vi "RAWFileLoadSample.vi"() -> ()   [LabVIEW 8.6]
panel:
  in  "Stop":bool
  out "Picture":picture
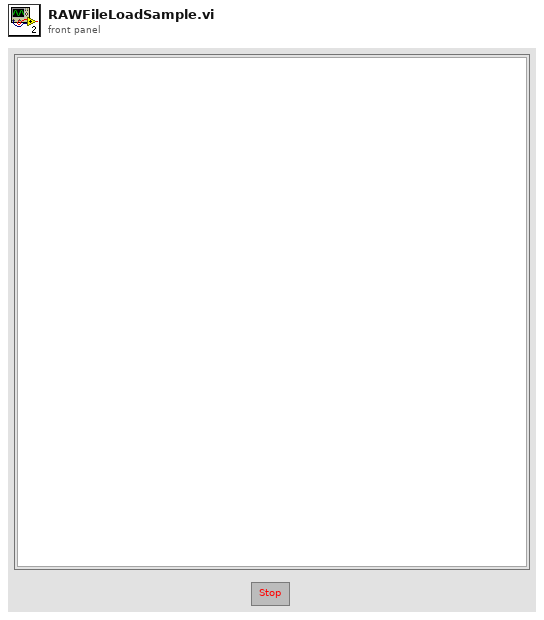
[diagram p1: front panel]
types:
  T1 = typedef "LVBoundsTypeDef.ctl" = cluster{"Width":u32, "Height":u32}
  T2 = cluster{"Width":i32, "Height":i32, "Byte Per Line":i32, "Real Bit Per Pixel":u16, "Interleave":i32}
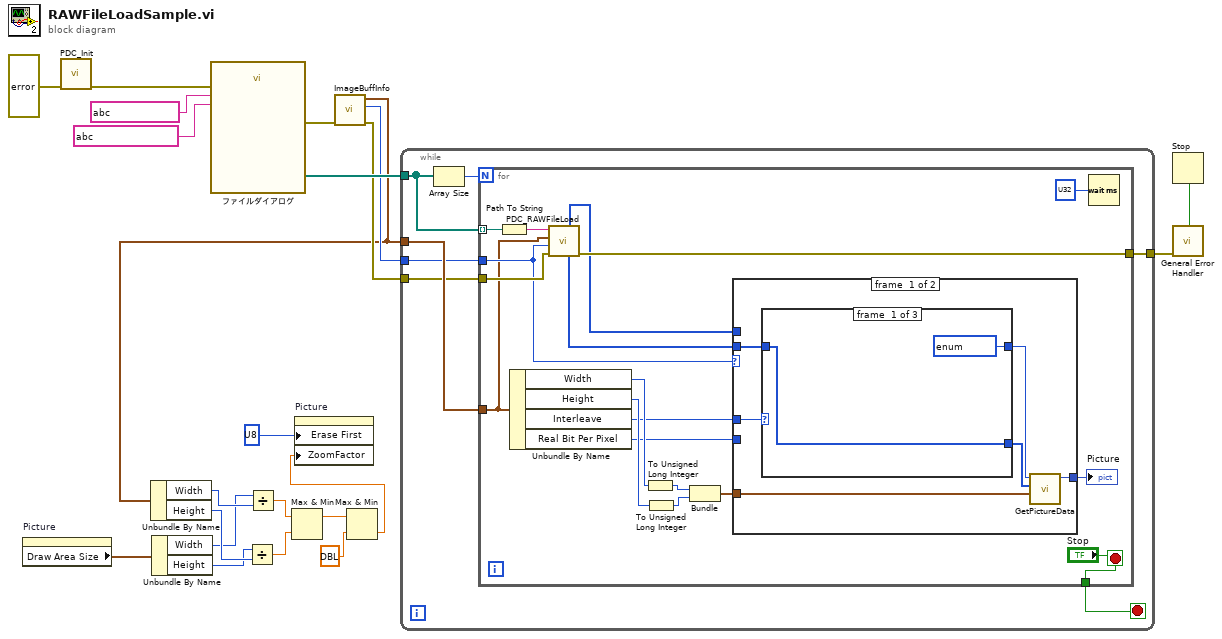
[diagram p0: block diagram]
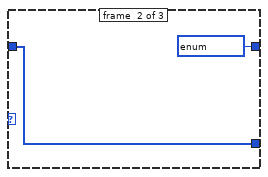
[diagram p2: hidden frame]
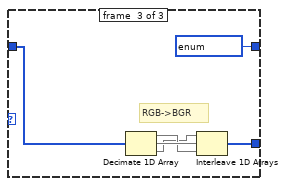
[diagram p3: hidden frame]
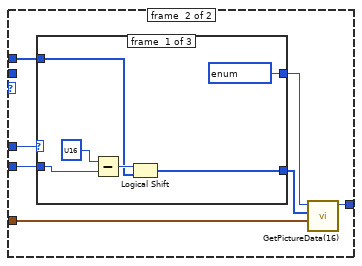
[diagram p4: hidden frame]
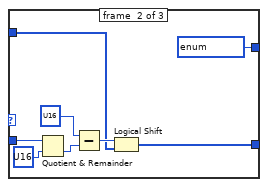
[diagram p5: hidden frame]
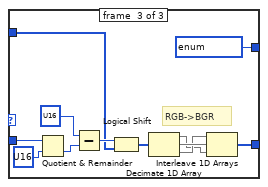
[diagram p6: hidden frame]
diagram:
  n1 = property on="Picture" class="Pict"() -> ("Draw Area Size"=w3:T1)  [unwired: 2 in, 2 out]
  n2 = call "PDC_Init.vi"("error in (no error)"=errorcluster ?) -> ("error out"=w19:errorcluster)  [unwired: 8 in, 2 out]
  n3 = Unbundle By Name(w3) -> ("Width"=w9:u32, "Height"=w8:u32)
  n4 = call "ファイルダイアログ"("error in"=w19, "pattern (all files)"=string ?, "pattern label"=string ?) -> ("selected paths"=w17:path[], "error out"=w16:errorcluster)  [unwired: 9 in, 2 out]
  n5 = call "ImageBuffInfo.vi"("error in (no error)"=w16) -> ("error out"=w14:errorcluster, "Raw Bit Depth"=w15:u32, "Image Buff Info"=w2:T2)  [unwired: 7 in, 1 out]
  n6 = Unbundle By Name(w2) -> ("Width"=w11:i32, "Height"=w10:i32)
  n7 = Divide(x=w8, y=w10) -> (x/y=w6:dbl)
  n8 = Divide(x=w9, y=w11) -> (x/y=w7:dbl)
  n9 = Max & Min(x=w7, y=w6) -> (max(x,y)=w5:dbl)  [unwired: 1 out]
  n10 = Max & Min(x=w5, y=dbl ?) -> (min(x,y)=w1:dbl)  [unwired: 1 out]
  n11 = property on="Picture" class="Pict"("Erase First"=u8 ? ("最初に削除"), "ZoomFactor"=w1) -> ()  [unwired: 2 in, 2 out]
  n12 = while {
    tunnel: w17 -> [w28]
    tunnel: w2 -> [w27]
    tunnel: w15 -> [w26]
    tunnel: w14 -> [w25]
    tunnel: [w24] -> w13
    stop <- w23 stop-if-true
    n13 = Array Size(array=w28) -> (size(s)=w29:i32)
    n14 = for {
      N: w29 -> [_]
      tunnel: w28 -> [w46] mode=indexing
      tunnel: w27 -> [w32]
      tunnel: w26 -> [w42]
      tunnel: w25 -> [w44]
      tunnel: [w43] -> w24
      tunnel: ["Stop"] -> w23
      stop <- "Stop" stop-if-true
      n15 = Path To String(path=w46) -> (string=w45:string)
      n16 = Unbundle By Name(w32) -> ("Width"=w37:i32, "Height"=w36:i32, "Interleave"=w31:i32, "Real Bit Per Pixel"=w30:u16)
      n17 = call "PDC_RAWFileLoad.vi"("FileName"=w45, "ImageBuffInfo"=w32, "RawBitDepth"=w42, "error in (no error)"=w44) -> ("Data(16Bit)"=w39:u16[], "Data(8Bit)"=w41:u8[], "error out"=w43:errorcluster)  [unwired: 2 in, 2 out]
      n18 = To Unsigned Long Integer(number=w37) -> (unsigned 32bit integer=w33:u32)
      n19 = To Unsigned Long Integer(number=w36) -> (unsigned 32bit integer=w35:u32)
      n20 = Bundle(w33, w35) -> (w38:cluster{u32, u32})  [unwired: 1 in]
      n21 = case shown="1..3, デフォルト" w42 {
        tunnel: w41 -> [w48 _]
        tunnel: [w52 w70] -> w40
        tunnel: w39 -> [_ w65]
        tunnel: w38 -> [w53 w69]
        tunnel: w31 -> [w49 w68]
        tunnel: w30 -> [_ w66]
        frame #0 {
          n22 = case shown="2" w49 {
            tunnel: [enum16{"MONO", "COLOR"} ? ("ColorType") enum16{"MONO", "COLOR"} ? ("ColorType") enum16{"MONO", "COLOR"} ? ("ColorType")] -> w50
            tunnel: [w54 w56 w62] -> w51
            tunnel: w48 -> [w54 w56 w61]
            frame #0 {
            }
            frame #1 {
            }
            frame #2 {
              # "RGB->BGR"
              n23 = Decimate 1D Array(w61) -> (w59:u8[], w60:u8[], w58:u8[])
              n24 = Interleave 1D Arrays(w58, w60, w59) -> (w62:u8[])
            }
          }
          n25 = call "GetPictureData.vi"("Resolution"=w53, "Data(8Bit)"=w51, "ColorType"=w50) -> ("new picture"=w52:picture)  [unwired: 4 in]
        }
        frame #1 {
          n26 = case shown="2" w68 {
            tunnel: [enum16{"MONO", "COLOR"} ? ("ColorType") enum16{"MONO", "COLOR"} ? ("ColorType") enum16{"MONO", "COLOR"} ? ("ColorType")] -> w67
            tunnel: w66 -> [w73 w79 w92]
            tunnel: w65 -> [w74 w81 w90]
            tunnel: [w71 w77 w88] -> w64
            frame #0 {
              n27 = Subtract(x=u16 ?, y=w73) -> (x-y=w75:u16)
              n28 = Logical Shift(y=w75, x=w74) -> (x << y=w71:u16[])
            }
            frame #1 {
              n29 = Quotient & Remainder(x=w79, y=u16 ?) -> (floor(x/y)=w80:u16)  [unwired: 1 out]
              n30 = Subtract(x=u16 ?, y=w80) -> (x-y=w82:u16)
              n31 = Logical Shift(y=w82, x=w81) -> (x << y=w77:u16[])
            }
            frame #2 {
              # "RGB->BGR"
              n32 = Quotient & Remainder(x=w92, y=u16 ?) -> (floor(x/y)=w93:u16)  [unwired: 1 out]
              n33 = Subtract(x=u16 ?, y=w93) -> (x-y=w94:u16)
              n34 = Logical Shift(y=w94, x=w90) -> (x << y=w89:u16[])
              n35 = Decimate 1D Array(w89) -> (w85:u16[], w87:u16[], w86:u16[])
              n36 = Interleave 1D Arrays(w86, w87, w85) -> (w88:u16[])
            }
          }
          n37 = call "GetPictureData(16).vi"("Resolution"=w69, "Data(16Bit)"=w64, "ColorType"=w67) -> ("new picture"=w70:picture)  [unwired: 4 in]
        }
      }
      "Picture" <- w40
      n38 = Wait (ms)(milliseconds to wait=u32 ? ("ミリ秒待機時間")) -> ()  [unwired: 1 out]
    }
  }
  n39 = call <vilib>:"General Error Handler.vi"("error in (no error)"=w13) -> ("error?"=w18:bool)  [unwired: 10 in, 4 out]
  n40 = Stop(stop? (T)=w18) -> ()
